vi "Drive.vi"() -> ()   [LabVIEW 2012]
uses:
  State_Machine_Enum.ctl
  Robot Global Data.vi
  <vilib>/Rock Robotics/WPI/RobotDrive/WPI_RobotDriveGetSetRefNum.vi
panel:
  out "Loop Difference":u32
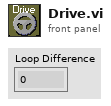
[diagram p1: front panel]
types:
  T1 = typedef "State_Machine_Enum.ctl" = enum16{"Init", "Idle", "Start", "Do", "Stop"}
  T2 = typedef "WPI_RobotDriveDevRef.ctl" = cluster{"DevStatus":errorcluster, "Motors[]":T3[], "Square Inputs":bool, "Max Output":dbl, "Isochronous":bool}
  T3 = typedef "WPI_MotorControlDeviceRef.ctl" = cluster{"DeviceStatus":errorcluster, "Type":enum16{"PWM", "CAN"}, "PWM":cluster{"Digital Module":T4, "PWM Channel":T5, "DeadBand":T6}, "CAN":cluster{"Device Number":u8, "Control Mode":T7, "Semaphore":T8, "Max Vout":dbl}, "Invert":bool, "TransformRef":T9, "InvTransformRef":T9}
  T4 = typedef "FPGA_TypedefDigitalModule.ctl" = enum16{"Digital Module 1", "Digital Module 2"}
  T5 = typedef "FPGA_DIOPWMChannel.ctl" = enum8{"PWM 1", "PWM 2", "PWM 3", "PWM 4", "PWM 5", "PWM 6", "PWM 7", "PWM 8", "PWM 9", "PWM 10", "Invalid"}
  T6 = typedef "WPI_PWMDeadband.ctl" = cluster{"Name":string, "maxPositivePwm":i32, "minPositivePwm":i32, "centerPwm":i32, "maxNegativePwm":i32, "minNegativePwm":i32, "angularRange":u16}
  T7 = typedef "WPI_CANJaguar_ControlMode.ctl" = enum8{"Percent VBus", "Current", "Speed", "Position", "Voltage"}
  T8 = typedef "Semaphore RefNum" = refnum<k1>
  T9 = typedef "WPI_PWMTransform_ConPane.ctl" = refnum<vi>
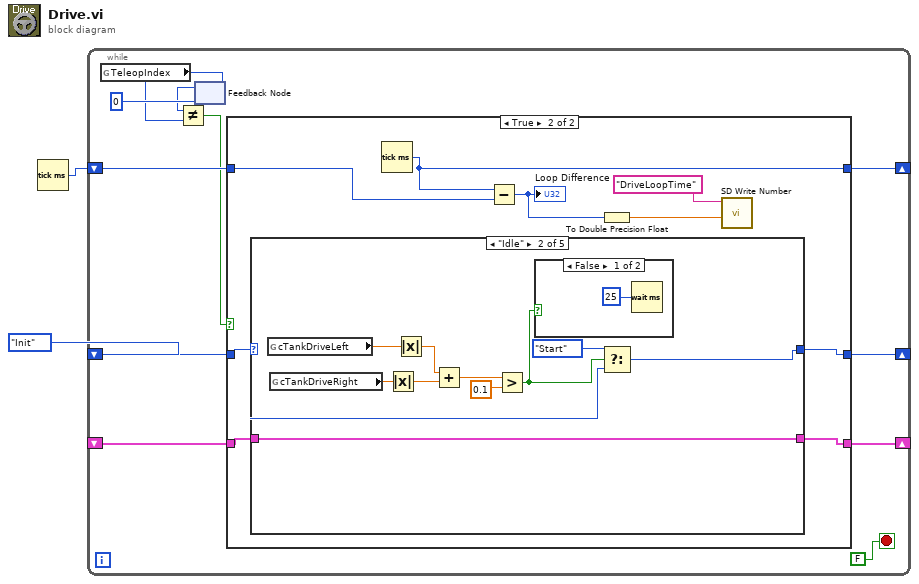
[diagram p0: block diagram]
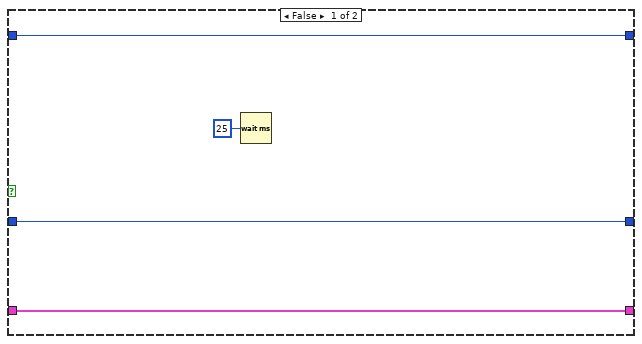
[diagram p2: hidden frame]
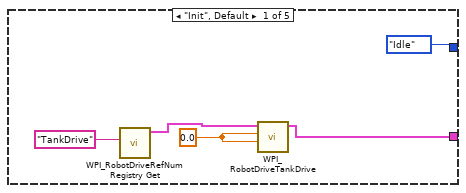
[diagram p3: hidden frame]
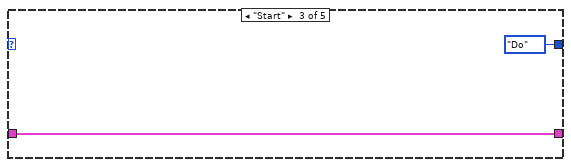
[diagram p5: hidden frame]
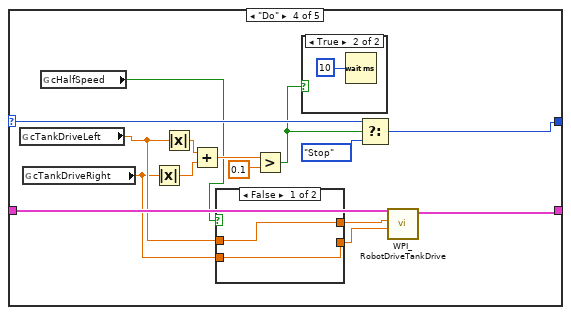
[diagram p6: hidden frame]
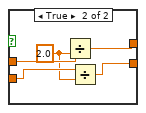
[diagram p7: hidden frame]
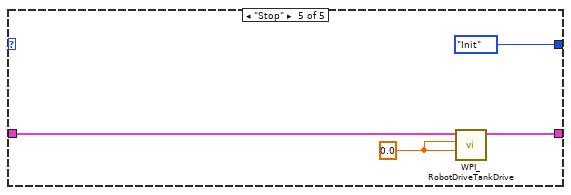
[diagram p9: hidden frame]
diagram:
  n1 = Tick Count (ms)() -> (millisecond timer value=w1:u32)
  n2 = while {
    shift-right: [w12] -> _
    shift-left: State_Machine_Enum."Init" ("State") -> [w13]
    shift-right: [w11] -> _
    shift-left: _ -> [w10]
    shift-right: [w8] -> _
    shift-left: w1 -> [w9]
    stop <- FALSE stop-if-true
    n3 = global read "Robot Global Data.vi" "TeleopIndex"() -> (w5:i32)
    n4 = feedback #1(0 ("TeleopIndex")) -> (w4:i32)
    n5 = Not Equal?(x=w4, y=w5) -> (x != y?=w3:bool)
    n6 = feedback-in #1(w5) -> ()
    n7 = case shown="True" w3 {
      tunnel: w13 -> [w16 w26]
      tunnel: [w16 w25] -> w12
      tunnel: [w15 w24] -> w11
      tunnel: w10 -> [w15 w23]
      tunnel: w9 -> [w17 w22]
      tunnel: [w17 w21] -> w8
      frame False {
        n8 = Wait (ms)(milliseconds to wait=u32 25) -> ()  [unwired: 1 out]
      }
      frame True {
        n9 = case shown="\"Idle\"" w26 {
          selector: w26 -> [_ w37 _ w56 _]
          tunnel: [State_Machine_Enum."Idle" ("State") w36 State_Machine_Enum."Do" ("State") w55 State_Machine_Enum."Init" ("State")] -> w25
          tunnel: [w28 w32 w45 w54 w71] -> w24
          tunnel: w23 -> [_ w32 w45 w51 w70]
          frame "Init", Default {
            w29 = 0.0 ("Left axis value")
            n10 = call <vilib>:"WPI_RobotDriveRefNum Registry Get.vi"("refnum name"="TankDrive") -> ("RobotDriveDevRef"=w27:T2)  [unwired: 9 in, 1 out]
            n11 = call <vilib>:"WPI_RobotDriveTankDrive.vi"("Right axis value"=w29, "Left axis value"=w29, "RobotDriveDevRef"=w27) -> ("RobotDriveDevRef"=w28:T2)  [unwired: 6 in, 2 out]
          }
          frame "Idle" {
            n12 = global read "Robot Global Data.vi" "cTankDriveLeft"() -> (w35:dbl)
            n13 = global read "Robot Global Data.vi" "cTankDriveRight"() -> (w34:dbl)
            n14 = Absolute Value(x=w34) -> (abs(x)=w41:dbl)
            n15 = Absolute Value(x=w35) -> (abs(x)=w42:dbl)
            n16 = Add(x=w42, y=w41) -> (x+y=w40:dbl)
            n17 = Greater?(x=w40, y=0.1) -> (0:w38:bool)
            n18 = case shown="False" w38 {
              frame False {
                n19 = Wait (ms)(milliseconds to wait=u32 25) -> ()  [unwired: 1 out]
              }
              frame True {
              }
            }
            n20 = Select(t=State_Machine_Enum."Start" ("State"), s=w38, f=w37) -> (s? t:f=w36:T1)
          }
          frame "Start" {
          }
          frame "Do" {
            n21 = global read "Robot Global Data.vi" "cTankDriveLeft"() -> (w50:dbl)
            n22 = global read "Robot Global Data.vi" "cTankDriveRight"() -> (w49:dbl)
            n23 = global read "Robot Global Data.vi" "cHalfSpeed"() -> (w46:bool)
            n24 = Absolute Value(x=w49) -> (abs(x)=w59:dbl)
            n25 = Absolute Value(x=w50) -> (abs(x)=w60:dbl)
            n26 = Add(x=w60, y=w59) -> (x+y=w57:dbl)
            n27 = case shown="False" w46 {
              tunnel: w50 -> [w62 w67]
              tunnel: w49 -> [w61 w66]
              tunnel: [w62 w64] -> w47
              tunnel: [w61 w63] -> w48
              frame False {
              }
              frame True {
                w65 = 2.0 ("y")
                n28 = Divide(x=w67, y=w65) -> (x/y=w64:dbl)
                n29 = Divide(x=w66, y=w65) -> (x/y=w63:dbl)
              }
            }
            n30 = Greater?(x=w57, y=0.1) -> (0:w53:bool)
            n31 = case shown="True" w53 {
              frame False {
              }
              frame True {
                n32 = Wait (ms)(milliseconds to wait=u32 10) -> ()  [unwired: 1 out]
              }
            }
            n33 = Select(t=w56, s=w53, f=State_Machine_Enum."Stop" ("State")) -> (s? t:f=w55:T1)
            n34 = call <vilib>:"WPI_RobotDriveTankDrive.vi"("Right axis value"=w48, "Left axis value"=w47, "RobotDriveDevRef"=w51) -> ("RobotDriveDevRef"=w54:T2)  [unwired: 6 in, 2 out]
          }
          frame "Stop" {
            w72 = 0.0 ("Left axis value")
            n35 = call <vilib>:"WPI_RobotDriveTankDrive.vi"("Right axis value"=w72, "Left axis value"=w72, "RobotDriveDevRef"=w70) -> ("RobotDriveDevRef"=w71:T2)  [unwired: 6 in, 2 out]
          }
        }
        n36 = Tick Count (ms)() -> (millisecond timer value=w21:u32)
        n37 = Subtract(x=w21, y=w22) -> (x-y=w20:u32)
        "Loop Difference" <- w20
        n38 = To Double Precision Float(number=w20) -> (double precision float=w19:dbl)
        n39 = call <vilib>:"SD Write Number.vi"("Numeric"=w19, "Name"="DriveLoopTime") -> ()  [unwired: 8 in, 2 out]
      }
    }
  }
